vi "writeToXML.vi"(8 "error in (no error)":errorcluster, 10 "Class Label":string, 11 "PointingPositions in":refnum<class "PointingPositions.lvclass">) -> (0 "error out":errorcluster, 2 "XML out":string, 3 "PointingPositions out":refnum<class "PointingPositions.lvclass">)   [LabVIEW 2022 SP3, in "TCSDataDefinitions.lvlib" / "TCSPublicStatus.lvlib" / "PointingPositions.lvlib" / "PointingPositions.lvclass"]
uses:
  PointingPositions.lvclass
  PointingPositions.lvclass/PointingPositions.ctl
  AzElError/AzElError.lvclass
  TCSCommand/TargetConfiguration/Target/FixedTarget/AzElParameters/AzElParameters.lvclass
  CurrentTimes/ClockTimes/ClockTimes.lvclass
  TCSCommand/TargetConfiguration/Target/FixedTarget/RADecParameters/RADecParameters.lvclass
  CurrentRotatorPositions/CurrentRotatorPositions.lvclass
  RotatorPositions/RotatorPositions.lvclass
  <userlib>/Common/XML/XMLGenerator/XMLGenerator.lvclass
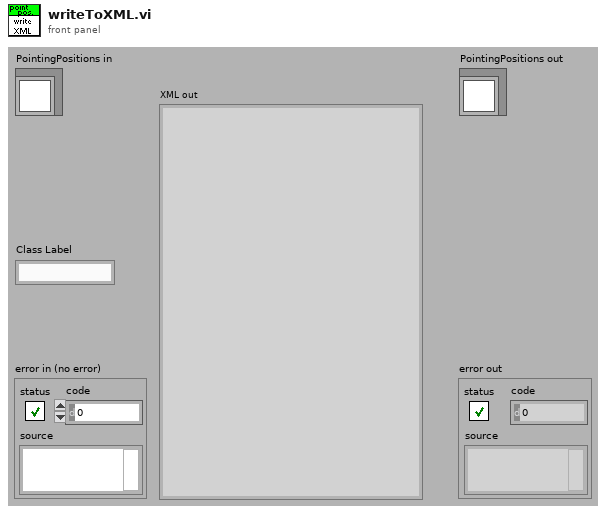
[diagram p1: front panel]
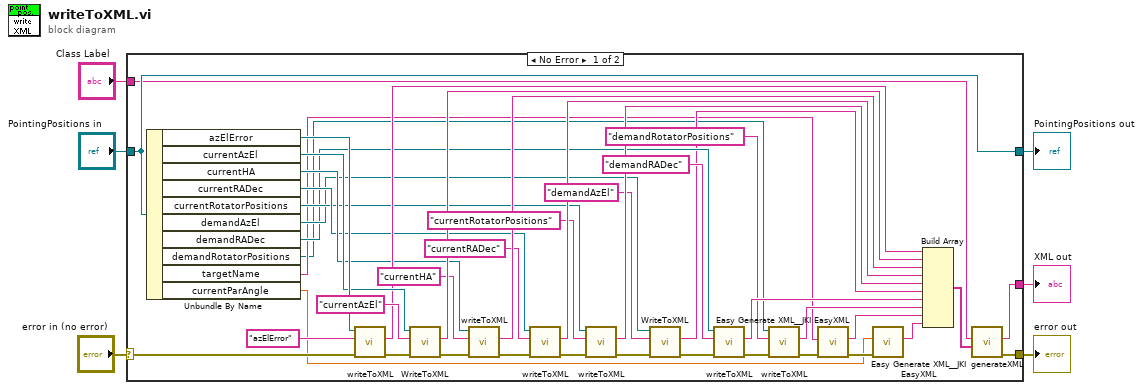
[diagram p0: block diagram]
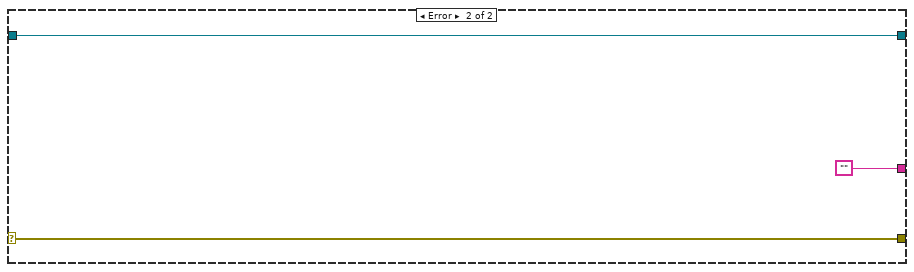
[diagram p2: hidden frame]
diagram:
  n1 = case shown="No Error" "error in (no error)" {
    selector: "error in (no error)" -> [w46 w52]
    tunnel: [w16 w52] -> w5
    tunnel: [w49 w51] -> w3
    tunnel: "PointingPositions in" -> [w49 w51]
    tunnel: [w17 ""] -> w2
    tunnel: "Class Label" -> [w11 _]
    frame No Error {
      n2 = Unbundle By Name(w49) -> ("azElError"=w48:refnum<class "AzElError.lvclass">, "currentAzEl"=w45:refnum<class "AzElParameters.lvclass">, "currentHA"=w40:refnum<class "ClockTimes.lvclass">, "currentRADec"=w35:refnum<class "RADecParameters.lvclass">, "currentRotatorPositions"=w32:refnum<class "CurrentRotatorPositions.lvclass">, "demandAzEl"=w27:refnum<class "AzElParameters.lvclass">, "demandRADec"=w25:refnum<class "RADecParameters.lvclass">, "demandRotatorPositions"=w10:refnum<class "RotatorPositions.lvclass">, "targetName"=w14:string, "currentParAngle"=w7:dbl)
      n3 = call-dynamic "writeToXML.vi"("error in (no error)"=w46, "Class Label"="azElError", "AzElError in"=w48) -> ("error out"=w43:errorcluster, "XML out"=w42:string)  [unwired: 6 in, 1 out]
      n4 = call-dynamic "WriteToXML.vi"("error in (no error)"=w43, "Class Label"="currentAzEl", "AzElParameters in"=w45) -> ("error out"=w37:errorcluster, "XML out"=w41:string)  [unwired: 6 in, 1 out]
      n5 = call-dynamic "writeToXML.vi"("error in (no error)"=w37, "Class Label"="currentHA", "ClockTimes in"=w40) -> ("error out"=w34:errorcluster, "XML out"=w38:string)  [unwired: 6 in, 1 out]
      n6 = call-dynamic "writeToXML.vi"("error in (no error)"=w34, "Class Label"="currentRADec", "RADecParameters in"=w35) -> ("error out"=w29:errorcluster, "XML out"=w33:string)  [unwired: 6 in, 1 out]
      n7 = call-dynamic "writeToXML.vi"("error in (no error)"=w29, "Class Label"="currentRotatorPositions", "CurrentRotatorPositions in"=w32) -> ("error out"=w26:errorcluster, "XML out"=w30:string)  [unwired: 6 in, 1 out]
      n8 = call-dynamic "WriteToXML.vi"("error in (no error)"=w26, "Class Label"="demandAzEl", "AzElParameters in"=w27) -> ("error out"=w23:errorcluster, "XML out"=w22:string)  [unwired: 6 in, 1 out]
      n9 = call-dynamic "writeToXML.vi"("error in (no error)"=w23, "Class Label"="demandRADec", "RADecParameters in"=w25) -> ("error out"=w19:errorcluster, "XML out"=w21:string)  [unwired: 6 in, 1 out]
      n10 = call-dynamic "writeToXML.vi"("error in (no error)"=w19, "Class Label"="demandRotatorPositions", "RotatorPositions in"=w10) -> ("error out"=w13:errorcluster, "XML out"=w15:string)  [unwired: 6 in, 1 out]
      n11 = call <vilib>:"Easy Generate XML__JKI EasyXML.vi"("error in (no error)"=w13, "LabVIEW Data"=w14) -> ("error out"=w9:errorcluster, "XML String"=w12:string)  [unwired: 8 in]
      n12 = call <vilib>:"Easy Generate XML__JKI EasyXML.vi"("error in (no error)"=w9, "LabVIEW Data"=w7) -> ("XML String"=w8:string)  [unwired: 8 in, 1 out]
      n13 = Build Array(w42, w41, w38, w33, w30, w22, w21, w15, w12, w8) -> (w18:string[])
      n14 = call <userlib>:"generateXML.vi"("childrenXML"=w18, "elementName"=w11) -> ("error out"=w16:errorcluster, "XML out"=w17:string)  [unwired: 7 in, 1 out]
    }
    frame Error {
    }
  }
  "error out" <- w5
  "PointingPositions out" <- w3
  "XML out" <- w2
